vi "Radio_Speed_Select.vi"(11 "Left Speed \nDemand\nPERCENT":T1=enum."Radio Selection 7") -> (3 "PERCENT":dbl)   [LabVIEW 2019]
uses:
  Radio_Speed_Ctrl.ctl
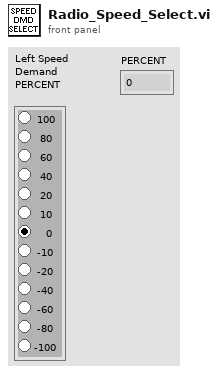
[diagram p1: front panel]
types:
  T1 = typedef "Radio_Speed_Ctrl.ctl" = enum32{"Radio Selection 1", "Radio Selection 2", "Radio Selection 3", "Radio Selection 4", "Radio Selection 5", "Radio Selection 6", "Radio Selection 7", "Radio Selection 8", "Radio Selection 9", "Radio Selection 10", "Radio Selection 11", "Radio Selection 12", "Radio Selection 13"}
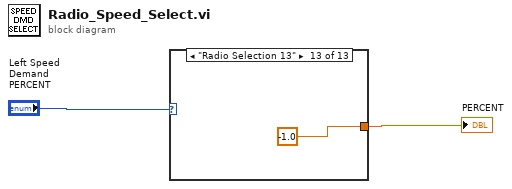
[diagram p0: block diagram]
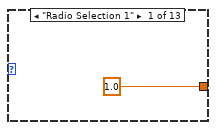
[diagram p2: hidden frame]
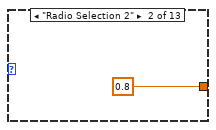
[diagram p3: hidden frame]
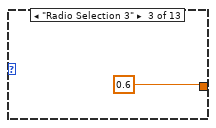
[diagram p4: hidden frame]
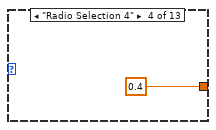
[diagram p5: hidden frame]
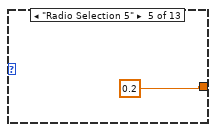
[diagram p6: hidden frame]
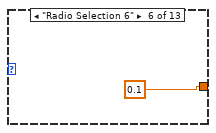
[diagram p7: hidden frame]
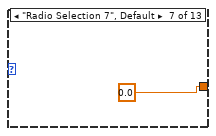
[diagram p8: hidden frame]
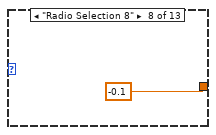
[diagram p9: hidden frame]
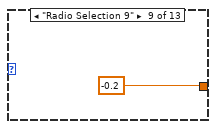
[diagram p10: hidden frame]
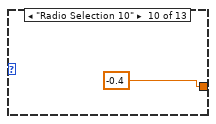
[diagram p11: hidden frame]
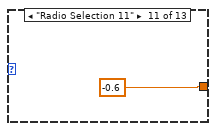
[diagram p12: hidden frame]
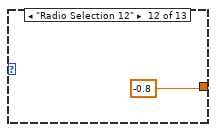
[diagram p13: hidden frame]
diagram:
  n1 = case shown="\"Radio Selection 13\"" "Left Speed \nDemand\nPERCENT" {
    tunnel: [1.0 0.8 0.6 0.4 0.2 0.1 0.0 -0.1 -0.2 -0.4 -0.6 -0.8 -1.0] -> w1
    frame "Radio Selection 1" {
    }
    frame "Radio Selection 2" {
    }
    frame "Radio Selection 3" {
    }
    frame "Radio Selection 4" {
    }
    frame "Radio Selection 5" {
    }
    frame "Radio Selection 6" {
    }
    frame "Radio Selection 7", Default {
    }
    frame "Radio Selection 8" {
    }
    frame "Radio Selection 9" {
    }
    frame "Radio Selection 10" {
    }
    frame "Radio Selection 11" {
    }
    frame "Radio Selection 12" {
    }
    frame "Radio Selection 13" {
    }
  }
  "PERCENT" <- w1
